vi "Set Digital Pin Mode.vi"(8 "Error In":errorcluster, 10 "Digtal Pin Modes":T1[](array[typedef]), 11 "LINX Device Config":T3) -> (0 "Error Out":errorcluster, 3 "LINX Device Config":T3)   [LabVIEW 2011, in "LVH-LINX.lvlib"]
doc: "Configure digital I/O pins as inputs or outputs."
uses:
  LVH-LINX.lvlib
  Private/Type Defs/LINX Device Config.ctl
  Private/Type Defs/Interface.ctl
  Private/Type Defs/TCP Config.ctl
  Private/Device/Type Defs/Digital Pin Mode Control.ctl
  Private/Device/Type Defs/Digital Pin Mode.ctl
  Private/Device/Error Type.ctl
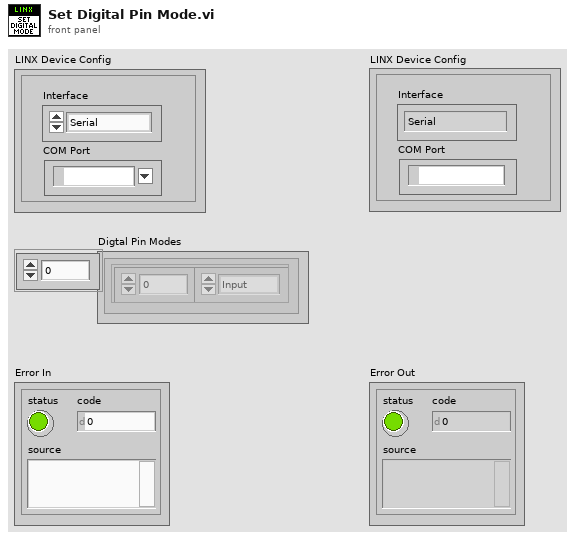
[diagram p1: front panel]
types:
  T1 = typedef "LVH-LINX.lvlib/Digital Pin Mode Control.ctl" = cluster{"Pin Number":u8, "Digital Pin Mode":T2}
  T2 = typedef "LVH-LINX.lvlib/Digital Pin Mode.ctl" = enum8{"Input", "Output"}
  T3 = typedef "LVH-LINX.lvlib/LINX Device Config.ctl" = cluster{"Interface":T4, "COM Port":refnum<visa-resource-name>, "Packet Number":u16, "TCP Configuration":T5}
  T4 = typedef "LVH-LINX.lvlib/Interface.ctl" = enum16{"Serial", "TCP"}
  T5 = typedef "LVH-LINX.lvlib/TCP Config.ctl" = cluster{"IP Address":string, "Port":dbl}
  T6 = typedef "LVH-LINX.lvlib/Error Type.ctl" = enum16{"Unknown", "Timeout", "Corrupt Return Packet", "Unable To Connect", "Command Not Supported"}
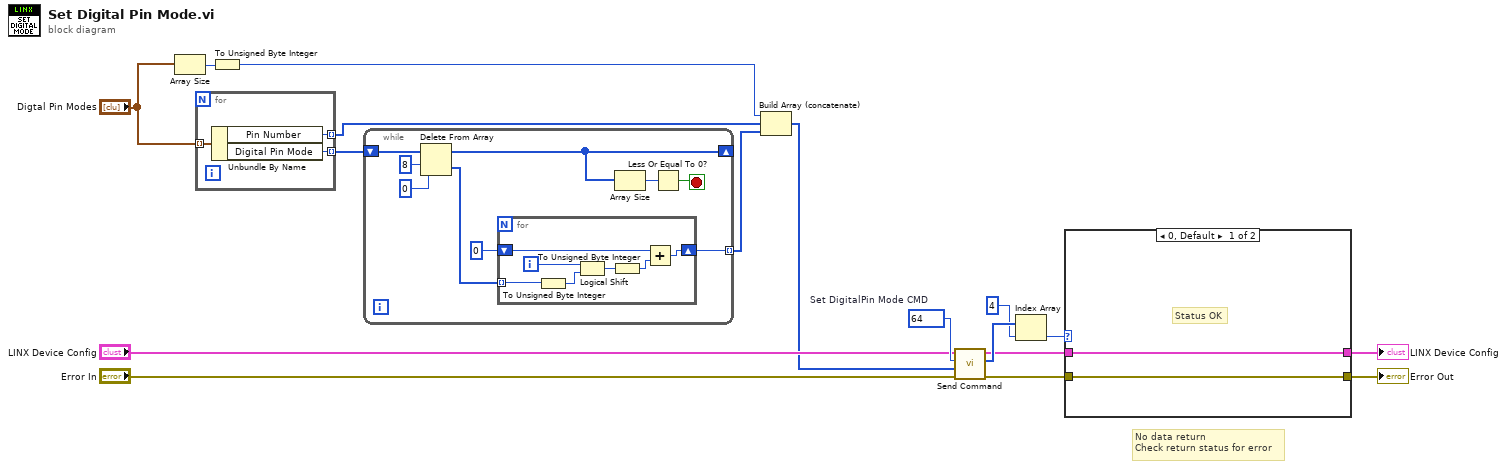
[diagram p0: block diagram]
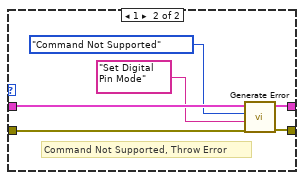
[diagram p2: hidden frame]
diagram:
  w16 = u16 64  # Set DigitalPin Mode CMD
  # "No data return\nCheck return status for error"
  n1 = Array Size(array="Digtal Pin Modes") -> (size(s)=w12:i32)
  n2 = for {
    tunnel: "Digtal Pin Modes" -> [w20] mode=indexing
    tunnel: [w19] -> w13 mode=indexing
    tunnel: [w18] -> w14 mode=indexing
    n3 = Unbundle By Name(w20) -> ("Pin Number"=w19:u8, "Digital Pin Mode"=w18:T2)
  }
  n4 = To Unsigned Byte Integer(number=w12) -> (unsigned 8bit integer=w11:u8)
  n5 = while {
    shift-right: [w26] -> _
    shift-left: w14 -> [w29]
    tunnel: [w21] -> w1 mode=indexing
    stop <- w24 stop-if-true
    n6 = Delete From Array(array=w29, length=8 ("index"), index=0 ("length")) -> (deleted portion=w22:T2[], array with subset deleted=w26:T2[])
    n7 = for {
      shift-right: [w35] -> w21
      shift-left: u8 0 ("y") -> [w36]
      tunnel: w22 -> [w32] mode=indexing
      i -> [w30]
      n8 = To Unsigned Byte Integer(number=w32) -> (unsigned 8bit integer=w31:u8)
      n9 = Logical Shift(y=w30, x=w31) -> (x << y=w34:u8)
      n10 = To Unsigned Byte Integer(number=w34) -> (unsigned 8bit integer=w33:u8)
      n11 = Add(x=w36, y=w33) -> (x+y=w35:u8)
    }
    n12 = Array Size(array=w26) -> (size(s)=w25:i32)
    n13 = Less Or Equal To 0?(x=w25) -> (x <= 0?=w24:bool)
  }
  n14 = Build Array (concatenate)(w11, w13, w1) -> (w10:u8[])
  n15 = call "Send Command.vi"("Error In"="Error In", "ARGS"=w10, "CMD"=w16, "LINX Device Config"="LINX Device Config") -> ("Error Out"=w3:errorcluster, "Packet"=w9:u8[], "LINX Device Config"=w5:T3)  [unwired: 5 in]
  n16 = Index Array(array=w9, index=4) -> (element=w7:u8)
  n17 = case shown="0, Default" w7 {
    tunnel: [w38 w41] -> w6
    tunnel: w5 -> [w38 w44]
    tunnel: [w37 w42] -> w4
    tunnel: w3 -> [w37 w43]
    frame 0, Default {
      # "Status OK"
    }
    frame 1 {
      # "Command Not Supported, Throw Error"
      n18 = call "Generate Error.vi"("Error In"=w43, "Arguments"="Set Digital Pin Mode", "Error Type"=Error_Type."Command Not Supported", "LINX Device Config"=w44) -> ("Error Out"=w42:errorcluster, "LINX Device Config"=w41:T3)  [unwired: 6 in]
    }
  }
  "Error Out" <- w4
  "LINX Device Config" <- w6
